vi "Modbus Master.vi"(7 "error in":errorcluster, 8 "Unit ID":u8=1, 9 "读取写入选择":string(combo), 10 "holding register values":u16[](array[numeric]) caption="写入保持寄存器的值", 11 "starting address":u16 caption="起始地址") -> (3 "register values":u16[](array[numeric]) caption="读取寄存器的值", 5 "error out":errorcluster)   [LabVIEW 2016]
uses:
  <vilib>/NI/Modbus Library/API/Modbus API.lvclass/Modbus API.ctl
  <vilib>/NI/Modbus Library/Transmission Data Unit/Transmission Data Unit.lvclass/Transmission Data Unit.ctl
  <vilib>/NI/Modbus Library/API/Master/Set Unit ID.vi
  <vilib>/NI/Modbus Library/Transmission Data Unit/Write Unit ID.vi
  <vilib>/NI/Modbus Library/API/Read Transmission Data Unit.vi
  <vilib>/NI/Modbus Library/API/Write Transmission Data Unit.vi
  <vilib>/NI/Modbus Library/API/master/Modbus Master.lvclass
  D:/Program Files (x86)/National Instruments/LabVIEW 2016/vi.lib/NI/Modbus Library/API/Modbus API.lvclass
  <vilib>/NI/Modbus Library/API/Wrapper/Create TCP Master.vi
  <vilib>/NI/Modbus Library/API/Wrapper/API Main.lvlib
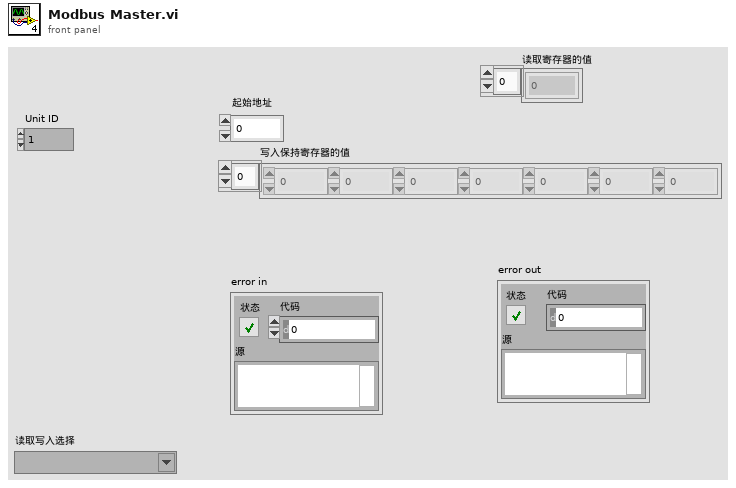
[diagram p1: front panel]
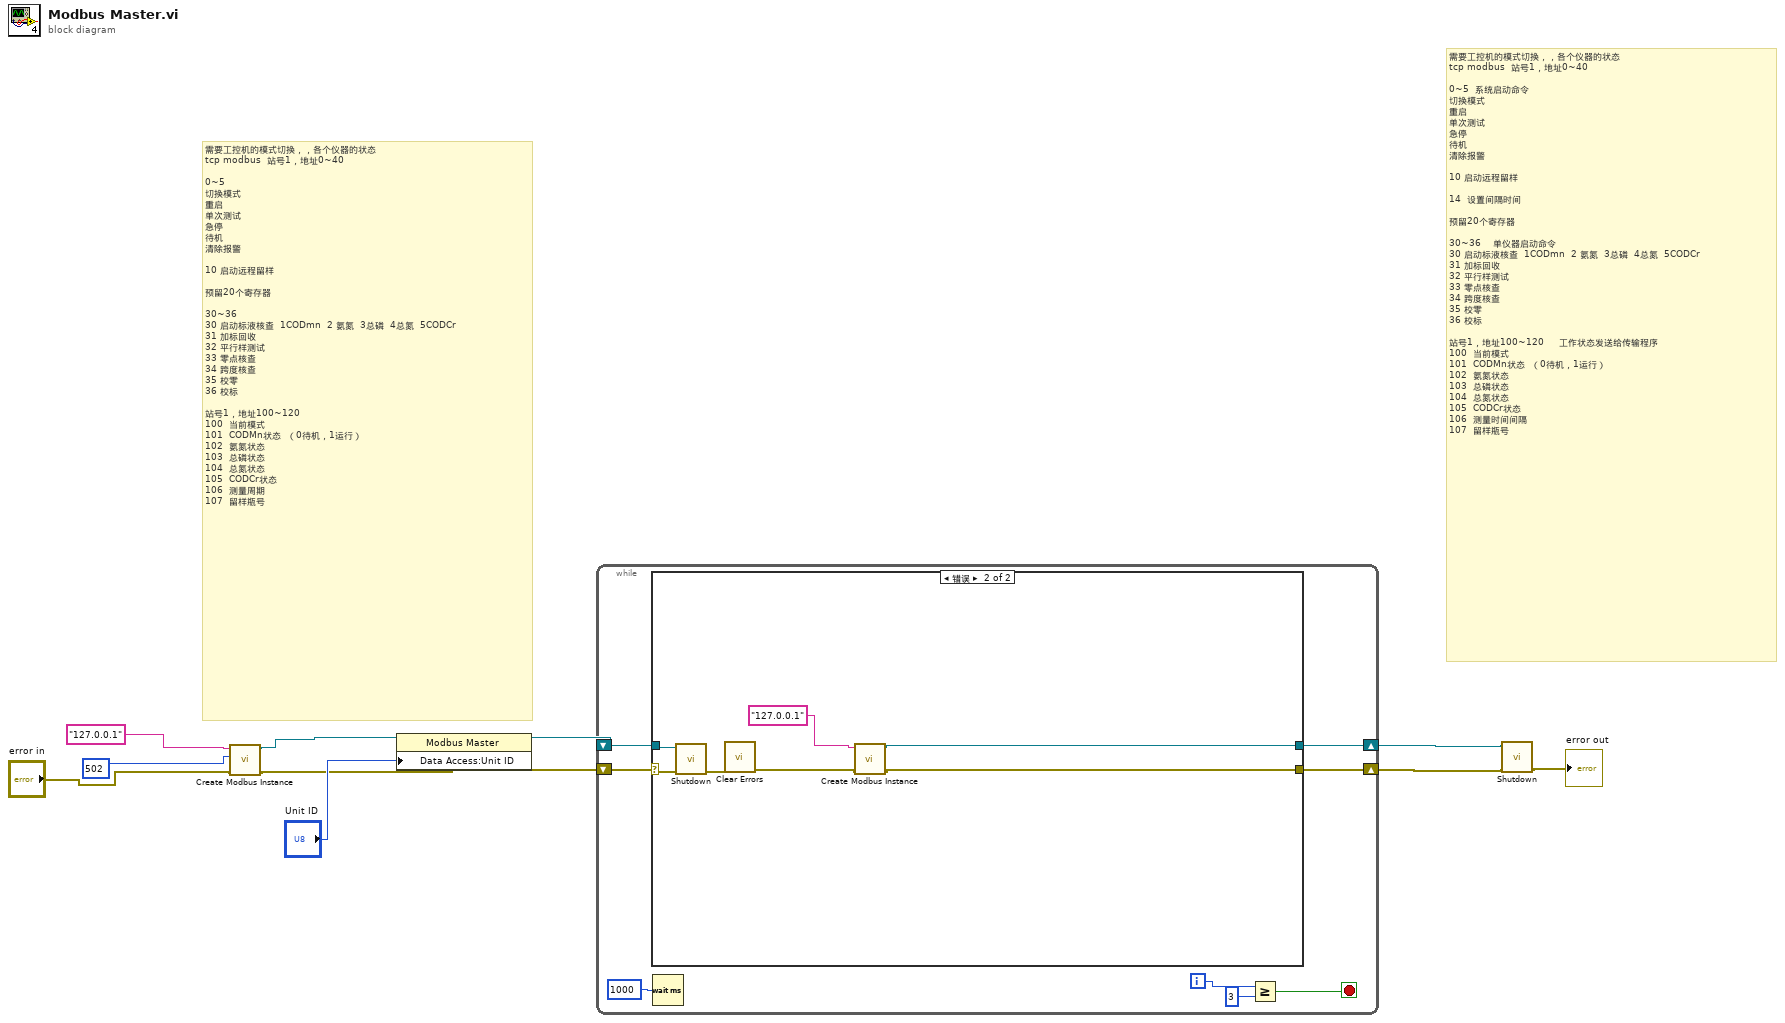
[diagram p0: block diagram]
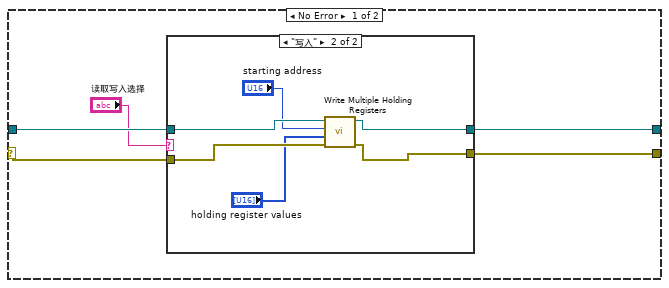
[diagram p2: hidden frame]
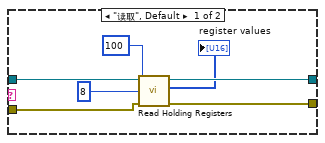
[diagram p3: hidden frame]
diagram:
  # "需要工控机的模式切换，，各个仪器的状态\ntcp modbus  站号1，地址0~40\n\n0~5  系统启动命令\n切换模式\n重启\n单次测试\n急停\n待机\n清除报警\n\n10 启动远程留样\n\n14  设置间隔时间\n\n预留20个寄存器\n\n30~36    单仪器启动命令\n30 启动标液核查  1CODmn  2 氨氮  3总磷  4总氮  5CODCr\n31 加标回收\n32 平行样测试\n33 零点核查\n34 跨度核查\n35 校零\n36 校标\n\n站号1，地址100~120     工作状态发送给传输程序\n100  当前模式\n101  CODMn状态  （0待机，1运行）\n102  氨氮状态\n103  总磷状态\n104  总氮状态\n105  CODCr状态\n106  测量时间间隔\n107  留样瓶号"
  # "需要工控机的模式切换，，各个仪器的状态\ntcp modbus  站号1，地址0~40\n\n0~5\n切换模式\n重启\n单次测试\n急停\n待机\n清除报警\n\n10 启动远程留样\n\n预留20个寄存器\n\n30~36\n30 启动标液核查  1CODmn  2 氨氮  3总磷  4总氮  5CODCr\n31 加标回收\n32 平行样测试\n33 零点核查\n34 跨度核查\n35 校零\n36 校标\n\n站号1，地址100~120\n100  当前模式\n101  CODMn状态  （0待机，1运行）\n102  氨氮状态\n103  总磷状态\n104  总氮状态\n105  CODCr状态\n106  测量周期\n107  留样瓶号"
  n1 = call-poly <vilib>:"Create Modbus Instance.vi"("error in"="error in", "port (502)"=u16 502, "address"="127.0.0.1") -> ("error out"=w4:errorcluster, "TCP master instance"=w5:refnum<class "Modbus Master.lvclass">)  [unwired: 7 in]
  n2 = property class="Modbus Master"(reference=w5, "Data Access:Unit ID"="Unit ID") -> (reference out=w10:refnum<class "Modbus Master.lvclass">)  [unwired: 1 in, 1 out]
  n3 = while {
    shift-right: [w16] -> w2
    shift-left: w4 -> [w15]
    shift-right: [w17] -> w3
    shift-left: w10 -> [w18]
    i -> [w13]
    stop <- w11 stop-if-true
    n4 = case shown="错误" w15 {
      selector: w15 -> [w20 w37]
      tunnel: w18 -> [w23 w39]
      tunnel: [w22 w41] -> w17
      tunnel: [w21 w40] -> w16
      frame No Error {
        n5 = case shown="\"写入\"" "读取写入选择" {
          tunnel: w23 -> [w30 w36]
          tunnel: [w28 w35] -> w22
          tunnel: [w27 w34] -> w21
          tunnel: w20 -> [w29 w33]
          frame "读取", Default {
            n6 = call-dynamic "Read Holding Registers.vi"("error in"=w29, "number of inputs"=u16 8 ("number of holding registers"), "starting address"=u16 100, "Modbus master in"=w30) -> ("error out"=w27:errorcluster, "register values"=→"register values":u16[], "Modbus master out"=w28:refnum<class "Modbus Master.lvclass">)  [unwired: 5 in]
          }
          frame "写入" {
            n7 = call-dynamic "Write Multiple Holding Registers.vi"("error in"=w33, "registers to write"="holding register values", "starting address"="starting address", "Modbus master in"=w36) -> ("error out"=w34:errorcluster, "Modbus master out"=w35:refnum<class "Modbus Master.lvclass">)  [unwired: 6 in]
          }
        }
      }
      frame Error {
        n8 = call-dynamic "Shutdown.vi"("error in"=w37, "Modbus master in"=w39) -> ("error out"=w38:errorcluster)  [unwired: 9 in]
        n9 = call <vilib>:"Clear Errors.vi"("error in (no error)"=w38) -> ("error out"=w42:errorcluster)  [unwired: 5 in, 1 out]
        n10 = call-poly <vilib>:"Create Modbus Instance.vi"("error in"=w42, "address"="127.0.0.1") -> ("error out"=w40:errorcluster, "TCP master instance"=w41:refnum<class "Modbus Master.lvclass">)  [unwired: 8 in]
      }
    }
    n11 = Wait (ms)(milliseconds to wait=u32 1000 ("等待时间（毫秒）")) -> ()  [unwired: 1 out]
    n12 = Greater Or Equal?(x=w13, y=3) -> (x >= y?=w11:bool)
  }
  n13 = call-dynamic "Shutdown.vi"("error in"=w2, "Modbus master in"=w3) -> ("error out"=→"error out":errorcluster)  [unwired: 9 in]
